vi "U Boat decode controller 2.vi"(3 "Main sheet In":u16=1500, 4 "Rudder In":u16=1500, 5 "Jib Sheet In":u16=1500, 6 "Manual In":i32[](array[numeric])) -> (0 "Main sheet Out":u16, 1 "Rudder Out":u16=1500, 2 "Jib Steet Out":u16)   [LabVIEW 2013]
doc: "This VI takes in the axis information from a Logitech F310 Game controller and outputs the values for the Jib sheet, Main sheet, and Rudder servos."
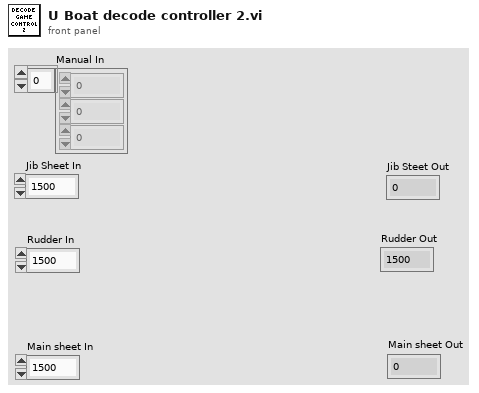
[diagram p1: front panel]
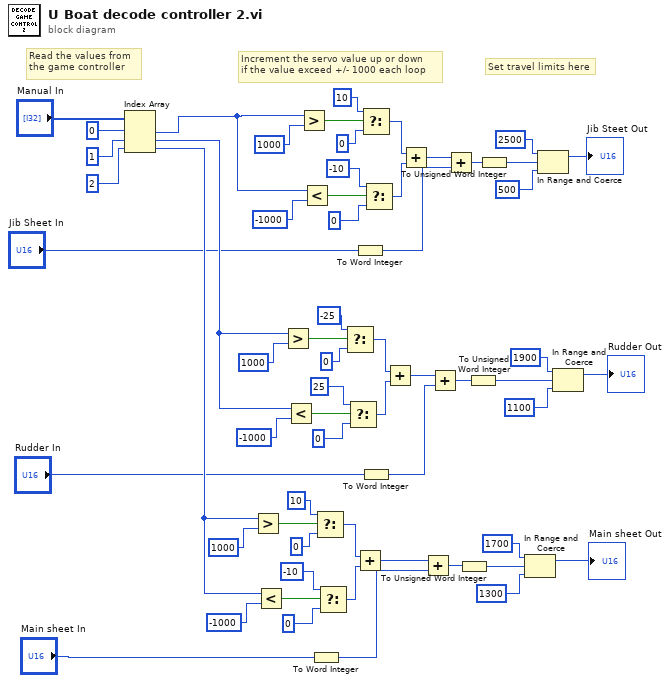
[diagram p0: block diagram]
diagram:
  # "Set travel limits here"
  # "Increment the servo value up or down\nif the value exceed +/- 1000 each loop"
  # "Read the values from\nthe game controller"
  n1 = Index Array(array="Manual In", index #1=0 ("index"), index #2=1 ("index"), index #3=2 ("index")) -> (element #1=w30:i32, element #2=w6:i32, element #3=w29:i32)
  n2 = Greater?(x=w29, y=1000) -> (0:w58:bool)
  n3 = Less?(x=w29, y=-1000) -> (x < y?=w54:bool)
  n4 = Greater?(x=w6, y=1000) -> (0:w10:bool)
  n5 = Less?(x=w6, y=-1000) -> (x < y?=w14:bool)
  n6 = Greater?(x=w30, y=1000) -> (0:w40:bool)
  n7 = Less?(x=w30, y=-1000) -> (x < y?=w44:bool)
  n8 = To Word Integer(number="Main sheet In") -> (16bit integer=w50:i16)
  n9 = Select(t=i16 10, s=w58, f=i16 0) -> (s? t:f=w53:i16)
  n10 = Select(t=i16 -10, s=w54, f=i16 0) -> (s? t:f=w52:i16)
  n11 = Select(t=i16 -25, s=w10, f=i16 0) -> (s? t:f=w15:i16)
  n12 = Select(t=i16 25, s=w14, f=i16 0) -> (s? t:f=w16:i16)
  n13 = To Word Integer(number="Jib Sheet In") -> (16bit integer=w37:i16)
  n14 = Add(x=w53, y=w52) -> (x+y=w51:i16)
  n15 = Select(t=i16 10, s=w40, f=i16 0) -> (s? t:f=w45:i16)
  n16 = To Word Integer(number="Rudder In") -> (16bit integer=w4:i16)
  n17 = Select(t=i16 -10, s=w44, f=i16 0) -> (s? t:f=w46:i16)
  n18 = Add(x=w15, y=w16) -> (x+y=w5:i16)
  n19 = Add(x=w45, y=w46) -> (x+y=w47:i16)
  n20 = Add(x=w51, y=w50) -> (x+y=w49:i16)
  n21 = Add(x=w5, y=w4) -> (x+y=w3:i16)
  n22 = Add(x=w47, y=w37) -> (x+y=w48:i16)
  n23 = To Unsigned Word Integer(number=w49) -> (unsigned 16bit integer=w18:u16)
  n24 = To Unsigned Word Integer(number=w3) -> (unsigned 16bit integer=w20:u16)
  n25 = To Unsigned Word Integer(number=w48) -> (unsigned 16bit integer=w22:u16)
  n26 = In Range and Coerce(upper limit=u16 1700, x=w18, lower limit=u16 1300) -> (coerced(x)=→"Main sheet Out":u16)  [unwired: 1 out]
  n27 = In Range and Coerce(upper limit=u16 2500, x=w22, lower limit=u16 500) -> (coerced(x)=→"Jib Steet Out":u16)  [unwired: 1 out]
  n28 = In Range and Coerce(upper limit=u16 1900, x=w20, lower limit=u16 1100) -> (coerced(x)=→"Rudder Out":u16)  [unwired: 1 out]
